vi "CréeTablePositionsGen.vi"(4 "IncFin (T)":bool=TRUE caption="Inclure\nPos Finale (T)", 6 "InvInt":bool caption="Interdire\nScan inverse", 8 "error in (no error)":errorcluster caption="entrée d'erreur (pas d'erreur)", 9 "Fin":dbl, 10 "Increment":dbl=1.0, 11 "Debut":dbl) -> (0 "error out":errorcluster caption="sortie d'erreur", 1 "nb pos":i32, 2 "Positions":dbl[](array[numeric]))   [LabVIEW 2019]
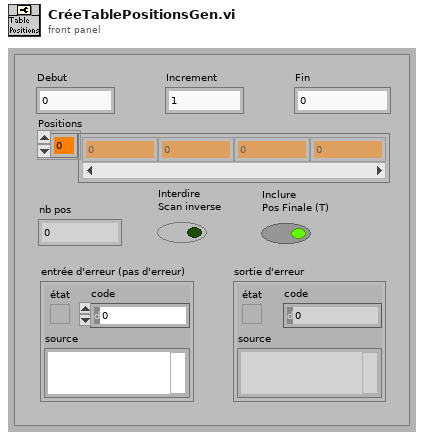
[diagram p1: front panel]
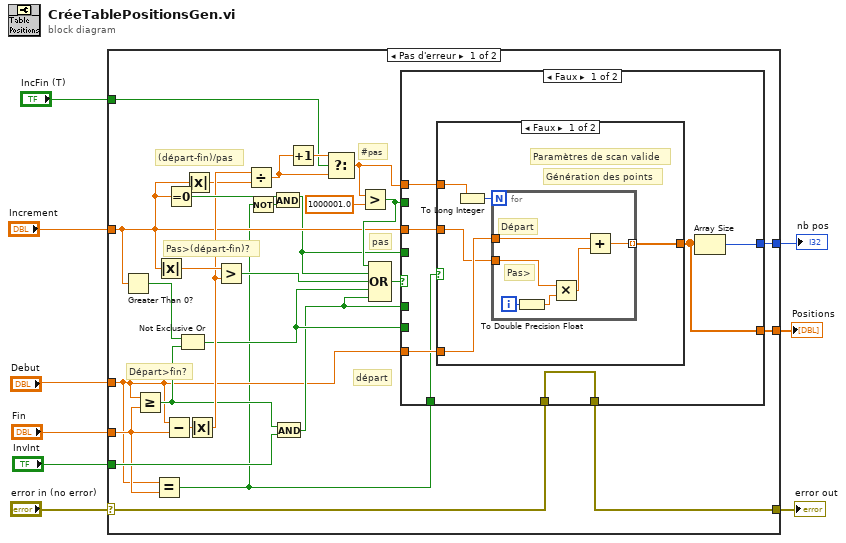
[diagram p0: block diagram]
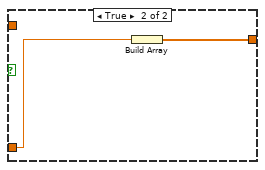
[diagram p2: hidden frame]
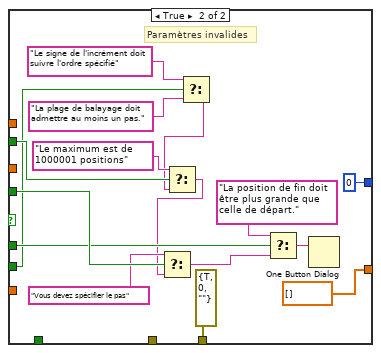
[diagram p3: hidden frame]
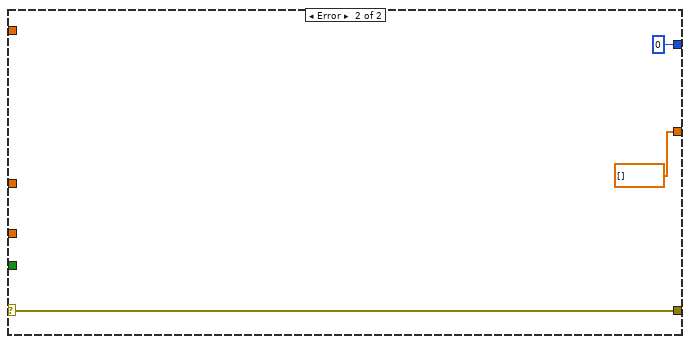
[diagram p4: hidden frame]
diagram:
  n1 = case shown="Pas d'erreur" "error in (no error)" {
    selector: "error in (no error)" -> [w29 w76]
    tunnel: "Fin" -> [w14 _]
    tunnel: "Debut" -> [w13 _]
    tunnel: "Increment" -> [w24 _]
    tunnel: [w31 0] -> w6
    tunnel: [w30 dbl[] []] -> w5
    tunnel: [w28 w76] -> w3
    tunnel: "InvInt" -> [w26 _]
    tunnel: "IncFin (T)" -> [w19 _]
    frame No Error {
      # "départ"
      # "pas"
      # "(départ-fin)/pas"
      # "#pas"
      # "Départ>fin?"
      # "Pas>(départ-fin)?"
      n2 = Greater Than 0?(x=w24) -> (x > 0?=w23:bool)
      n3 = Greater Or Equal?(x=w13, y=w14) -> (x >= y?=w22:bool)
      n4 = Equal?(x=w13, y=w14) -> (x = y?=w11:bool)
      n5 = Absolute Value(x=w24) -> (abs(x)=w35:dbl)
      n6 = Subtract(x=w13, y=w14) -> (x-y=w32:dbl)
      n7 = Equal To 0?(x=w24) -> (x = 0?=w37:bool)
      n8 = Not Exclusive Or(1:w22, 2:w23) -> (0:w18:bool)
      n9 = Absolute Value(x=w24) -> (abs(x)=w15:dbl)
      n10 = Absolute Value(x=w32) -> (abs(x)=w34:dbl)
      n11 = Greater?(x=w35, y=w34) -> (0:w36:bool)
      n12 = Divide(x=w34, y=w15) -> (x/y=w21:dbl)
      n13 = Not(x=w11) -> (.not. x?=w10:bool)
      n14 = And(x=w37, y=w10) -> (x .and. y?=w12:bool)
      n15 = And(x=w22, y=w26) -> (x .and. y?=w17:bool)
      n16 = Increment(x=w21) -> (x+1=w20:dbl)
      n17 = Select(t=w20, s=w19, f=w21) -> (s? t:f=w16:dbl)
      n18 = Greater?(x=w16, y=1000001.0) -> (0:w25:bool)
      n19 = Compound Arithmetic op=OR(w25, w12, w36, w18, w17) -> (w33:bool)
      n20 = case shown="Faux" w33 {
        tunnel: w17 -> [_ w70]
        tunnel: w13 -> [w44 _]
        tunnel: w16 -> [w42 _]
        tunnel: w24 -> [w43 _]
        tunnel: w12 -> [_ w71]
        tunnel: [w41 0] -> w31
        tunnel: [w38 dbl[] []] -> w30
        tunnel: w29 -> [w40 _]
        tunnel: [w40 errorcluster {"status"=TRUE, "code"=0, "source"=""} ("error IO")] -> w28
        tunnel: w25 -> [_ w65]
        tunnel: w18 -> [_ w62]
        tunnel: w11 -> [w39 _]
        frame False {
          n21 = case shown="Faux" w39 {
            tunnel: w44 -> [w48 w57]
            tunnel: w43 -> [w47 _]
            tunnel: w42 -> [w46 _]
            tunnel: [w45 w56] -> w38
            frame False {
              # "Paramètres de scan valide"
              # "Génération des points"
              n22 = To Long Integer(number=w46) -> (32bit integer=w49:i32)
              n23 = for {
                N: w49 -> [_]
                tunnel: [w52] -> w45 mode=indexing
                tunnel: w48 -> [w51]
                tunnel: w47 -> [w50]
                i -> [w55]
                # "Départ"
                # "Pas>"
                n24 = To Double Precision Float(number=w55) -> (double precision float=w54:dbl)
                n25 = Multiply(x=w50, y=w54) -> (x*y=w53:dbl)
                n26 = Add(x=w51, y=w53) -> (x+y=w52:dbl)
              }
            }
            frame True {
              n27 = Build Array(w57) -> (w56:dbl[])
            }
          }
          n28 = Array Size(array=w38) -> (size(s)=w41:i32)
        }
        frame True {
          # "Paramètres invalides"
          n29 = Select(t="Le signe de l'incrément doit suivre l'ordre spécifié", s=w62, f="La plage de balayage doit admettre au moins un pas.") -> (s? t:f=w60:string)
          n30 = Select(t="Le maximum est de 1000001 positions", s=w65, f=w60) -> (s? t:f=w59:string)
          n31 = Select(t="Vous devez spécifier le pas", s=w71, f=w59) -> (s? t:f=w58:string)
          n32 = Select(t="La position de fin doit être plus grande que celle de départ.", s=w70, f=w58) -> (s? t:f=w73:string)
          n33 = One Button Dialog(message=w73) -> ()  [unwired: 1 in, 1 out]
        }
      }
    }
    frame Error {
    }
  }
  "Positions" <- w5
  "error out" <- w3
  "nb pos" <- w6
